vi "Connect to LabJack.vi"(8 "Error In":errorcluster, 11 "Serial Number":string) -> (0 "Error Out":errorcluster, 3 "LabJack":refnum<k24>)   [LabVIEW 2018, in "ThorlabsLabJack.lvlib" / "ThorlabsLabJack.lvclass"]
uses:
  ThorlabsLabJack.lvclass
  C:/AME Test Engineering/LabVIEW/PPLs/Axis/Thorlabs/Thorlabs.MotionControl.IntegratedStepperMotorsCLI.dll
  PPLs/Axis/Thorlabs/Thorlabs.MotionControl.IntegratedStepperMotorsCLI.dll
  31e7e55e-c8ff-442e-97a5-577b4d87a9c2.vi
  d26ab8b0-f4e1-4565-b20b-125a1618cf4c.vi
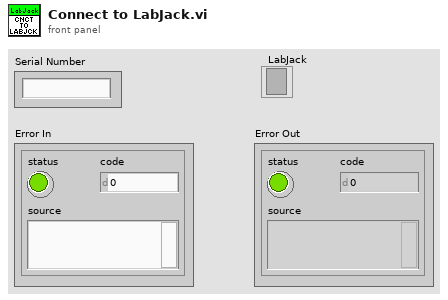
[diagram p1: front panel]
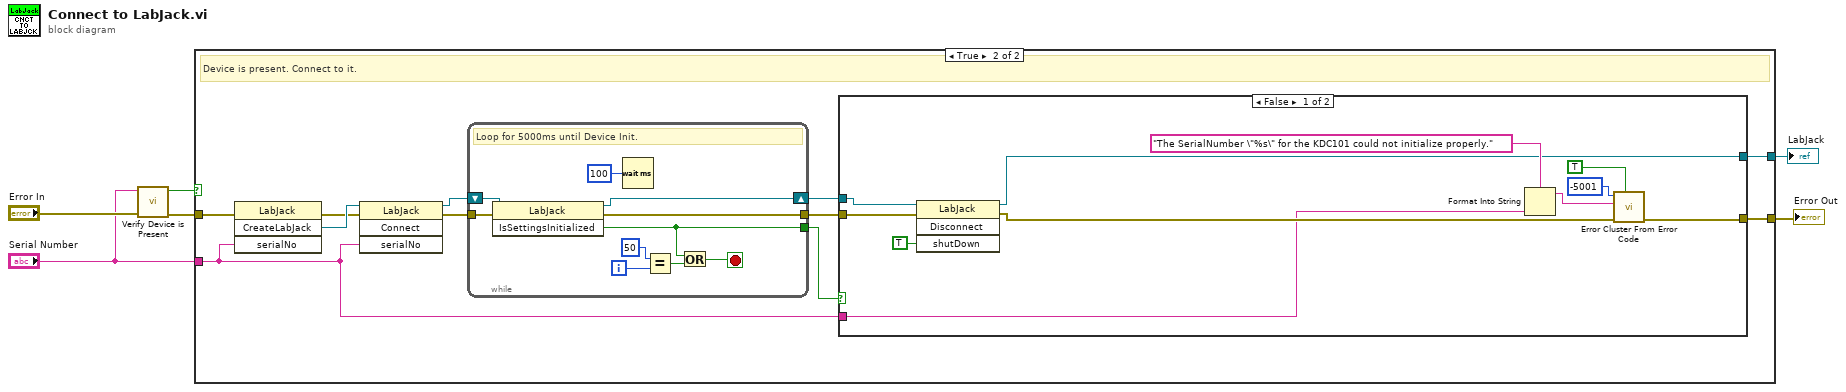
[diagram p0: block diagram]
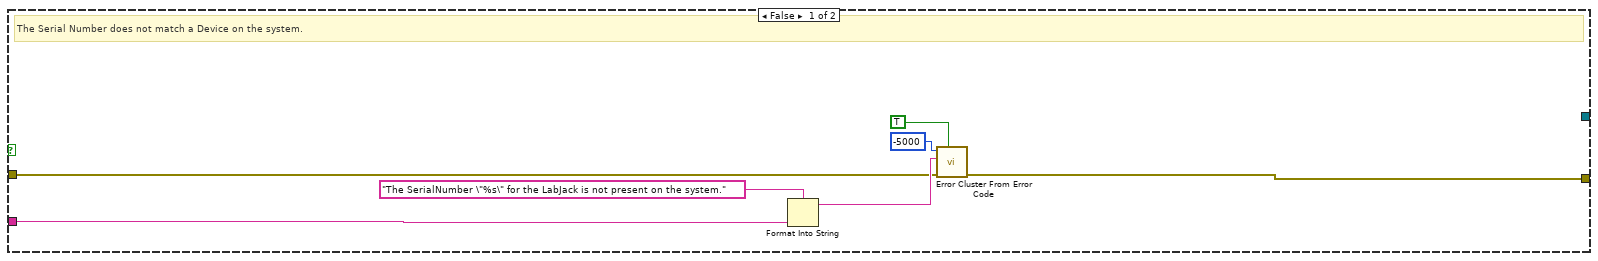
[diagram p2: hidden frame]
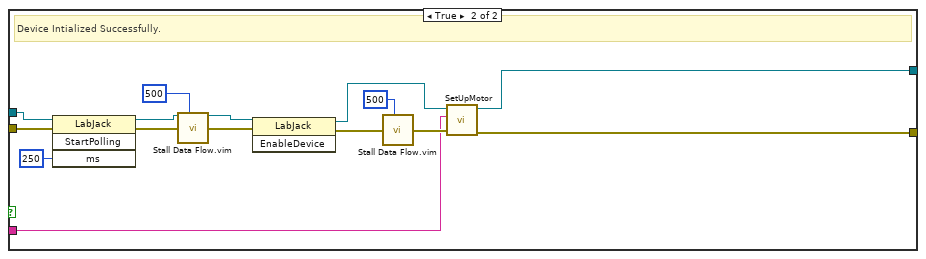
[diagram p3: hidden frame]
diagram:
  n1 = call "Verify Device is Present.vi"("Error In"="Error In", "Serial Number in"="Serial Number") -> ("Error Out"=w4:errorcluster, "Present?"=w5:bool)  [unwired: 8 in]
  n2 = case shown="True" w5 {
    tunnel: w4 -> [w9 w24]
    tunnel: "Serial Number" -> [w7 w16]
    tunnel: [w10 w15] -> w2
    tunnel: [_ w14] -> w1
    frame False {
      # "The Serial Number does not match a Device on the system."
      n3 = Format Into String(format string="The SerialNumber \"%s\" for the LabJack is not present on the system." ("error message (\"\")"), w7) -> (resulting string=w12:string)  [unwired: 2 in, 1 out]
      n4 = call <vilib>:"Error Cluster From Error Code.vi"("show call chain? (False)"=TRUE, "error in (no error)"=w9, "error message (\"\")"=w12, "error code (0)"=-5000) -> ("error out"=w10:errorcluster)  [unwired: 5 in]
    }
    frame True {
      # "Device is present. Connect to it."
      n5 = invoke class="LabJack" method="CreateLabJack"(error in=w24, "serialNo"=w16) -> (error out=w22:errorcluster, "CreateLabJack"=w23:refnum<k24>)  [unwired: 2 in, 2 out]
      n6 = invoke class="LabJack" method="Connect"(reference=w23, error in=w22, "serialNo"=w16) -> (reference out=w20:refnum<k24>, error out=w21:errorcluster)  [unwired: 1 in, 2 out]
      n7 = while {
        tunnel: w21 -> [w57]
        shift-right: [w51] -> w19
        shift-left: w20 -> [w58]
        tunnel: [w54] -> w18
        tunnel: [w50] -> w17
        i -> [w53]
        stop <- w52 stop-if-true
        # "Loop for 5000ms until Device Init."
        n8 = invoke class="LabJack" method="IsSettingsInitialized"(reference=w58, error in=w57) -> (reference out=w51:refnum<k24>, error out=w50:errorcluster, "IsSettingsInitialized"=w54:bool)  [unwired: 1 in]
        n9 = Wait (ms)(milliseconds to wait=u32 100) -> ()  [unwired: 1 out]
        n10 = Equal?(x=50, y=w53) -> (x = y?=w56:bool)
        n11 = Or(x=w54, y=w56) -> (x .or. y?=w52:bool)
      }
      n12 = case shown="False" w18 {
        tunnel: w19 -> [w34 w48]
        tunnel: w17 -> [w35 w49]
        tunnel: w16 -> [w25 w38]
        tunnel: [w28 w37] -> w15
        tunnel: [w26 w36] -> w14
        frame False {
          n13 = invoke class="LabJack" method="Disconnect"(reference=w34, error in=w35, "shutDown"=TRUE) -> (reference out=w26:refnum<k24>, error out=w27:errorcluster)  [unwired: 1 in, 2 out]
          n14 = Format Into String(format string="The SerialNumber \"%s\" for the KDC101 could not initialize properly." ("error message (\"\")"), w25) -> (resulting string=w31:string)  [unwired: 2 in, 1 out]
          n15 = call <vilib>:"Error Cluster From Error Code.vi"("show call chain? (False)"=TRUE, "error in (no error)"=w27, "error message (\"\")"=w31, "error code (0)"=-5001) -> ("error out"=w28:errorcluster)  [unwired: 5 in]
        }
        frame True {
          # "Device Intialized Successfully."
          n16 = invoke class="LabJack" method="StartPolling"(reference=w48, error in=w49, "ms"=250) -> (reference out=w43:refnum<k24>, error out=w46:errorcluster)  [unwired: 1 in, 2 out]
          n17 = call "Stall Data Flow.vim"("value in"=w46, "milliseconds to wait"=u32 500) -> ("value out"=w44:errorcluster)  [unwired: 1 out]
          n18 = invoke class="LabJack" method="EnableDevice"(reference=w43, error in=w44) -> (reference out=w39:refnum<k24>, error out=w41:errorcluster)  [unwired: 1 in, 1 out]
          n19 = call "Stall Data Flow.vim"("value in"=w41, "milliseconds to wait"=u32 500) -> ("value out"=w40:errorcluster)  [unwired: 1 out]
          n20 = call "SetUpMotor.vi"("Error In"=w40, "Serial Number"=w38, "LabJack in"=w39) -> ("Error Out"=w37:errorcluster, "reference out"=w36:refnum<k24>)  [unwired: 7 in]
        }
      }
    }
  }
  "Error Out" <- w2
  "LabJack" <- w1
